vi "MD420_ACT_TargetValue-LAPTOP-A1ILEVN9.vi"(0 "MD420.lvclass":refnum<class "MD420.lvclass">, 1 "SI656 PG 2nd Min in %":dbl, 2 "SI657 PG target SP":dbl, 3 "BC56 PUMA RELEB":bool, 4 "SI101 ACT 2nd Ctrl":dbl, 5 "error in (no error)":errorcluster, 6 "SI657 PG eff SP":dbl, 7 "ACT limit Setpoint":dbl) -> (14 "MD420.lvclass out":refnum<class "MD420.lvclass">, 16 "Outputs":T1, 19 "error out":errorcluster)   [LabVIEW 2022 SP3, in "MD420.lvclass"]
uses:
  MD420.lvclass
  MD420.lvclass/MD420.ctl
panel:
  in  "H 2":dbl=22.0 format="%#_13g"
  in  "Min":dbl=26.0 format="%#_13g"
  in  "Max":dbl=26.0 format="%#_13g"
  in  "H":dbl=22.0 format="%#_13g"
  # "MD420"
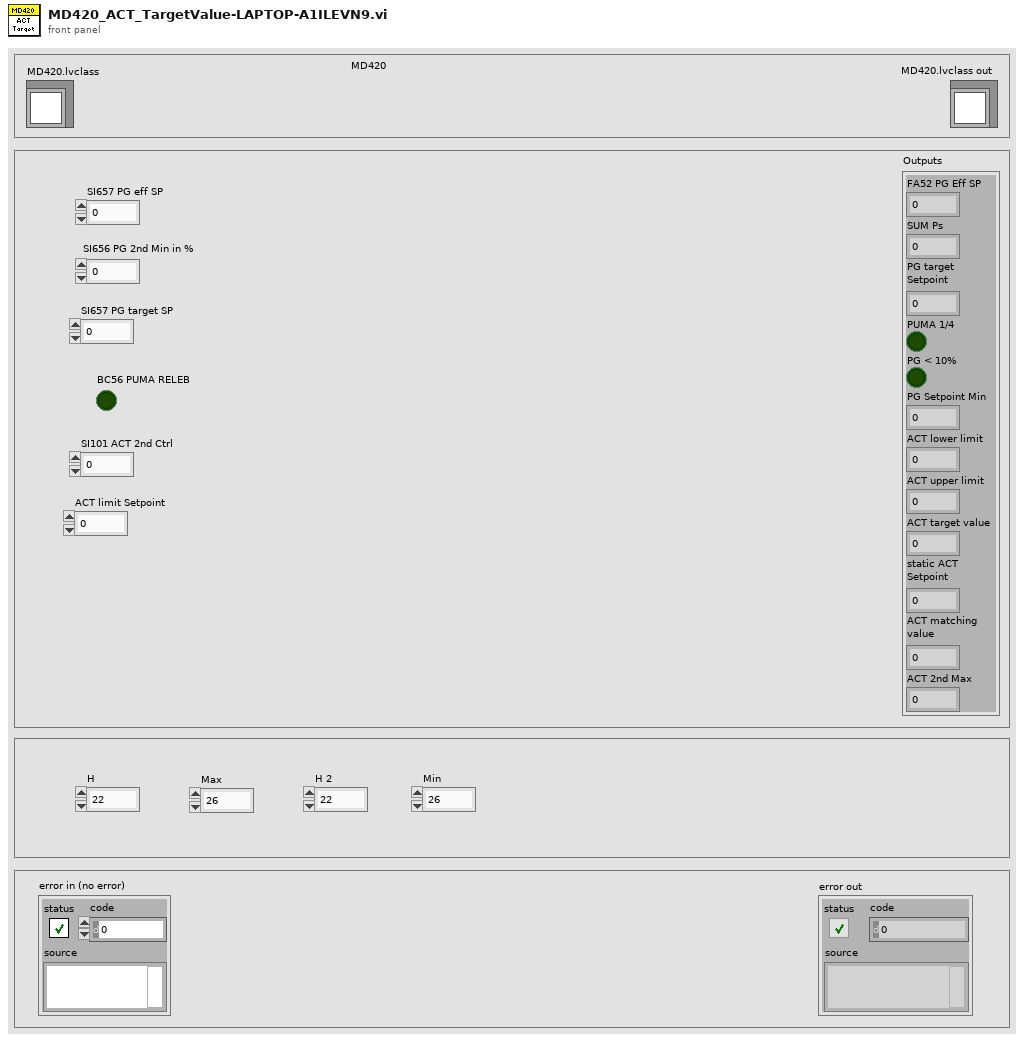
[diagram p1: front panel]
types:
  T1 = cluster{"FA52 PG Eff SP":dbl, "SUM Ps":dbl, "PG target\nSetpoint":dbl, "PUMA 1/4":bool, "PG < 10%":bool, "PG Setpoint Min":dbl, "ACT lower limit":dbl, "ACT upper limit":dbl, "ACT target value":dbl, "static ACT\nSetpoint":dbl, "ACT matching\nvalue":dbl, "ACT 2nd Max":dbl}
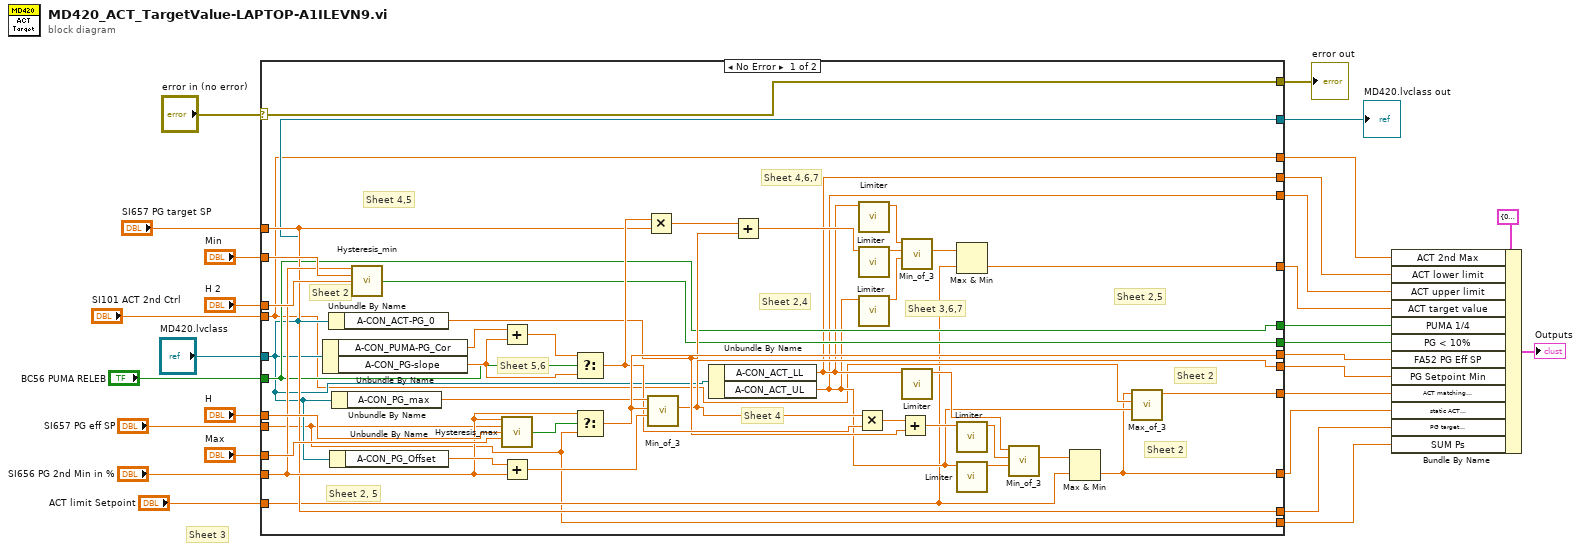
[diagram p0: block diagram]
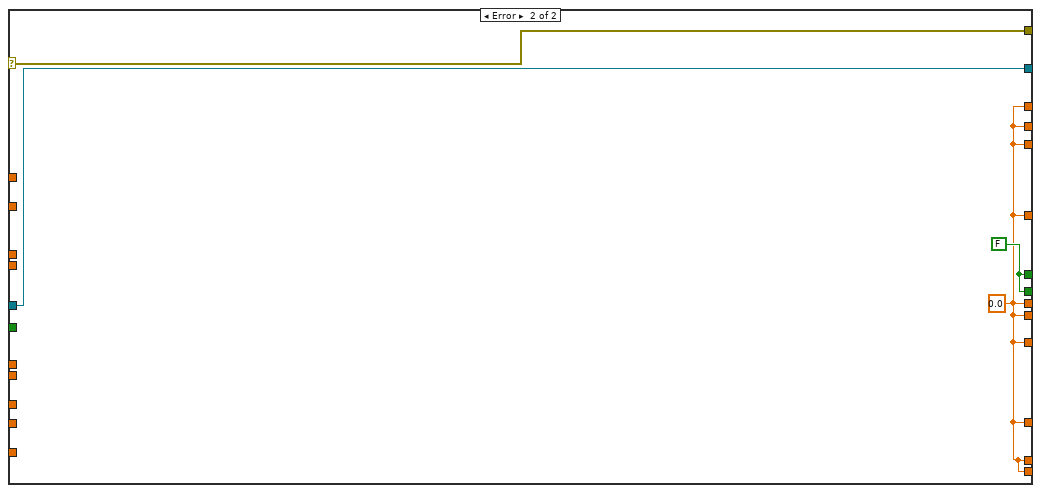
[diagram p2: hidden frame]
diagram:
  # "Sheet 3"
  n1 = case shown="No Error" "error in (no error)" {
    selector: "error in (no error)" -> [w69 w73]
    tunnel: [w69 w73] -> w27
    tunnel: "MD420.lvclass" -> [w47 w71]
    tunnel: "SI657 PG eff SP" -> [w29 _]
    tunnel: "SI656 PG 2nd Min in %" -> [w62 _]
    tunnel: "H" -> [w68 _]
    tunnel: "Max" -> [w67 _]
    tunnel: [w61 w70] -> w6
    tunnel: "Min" -> [w64 _]
    tunnel: "H 2" -> [w63 _]
    tunnel: "SI657 PG target SP" -> [w51 _]
    tunnel: "BC56 PUMA RELEB" -> [w50 _]
    tunnel: [w51 w70] -> w2
    tunnel: [w50 w72] -> w8
    tunnel: [w49 w72] -> w7
    tunnel: [w48 w70] -> w5
    tunnel: [w41 w70] -> w11
    tunnel: [w37 w70] -> w10
    tunnel: [w47 w71] -> w17
    tunnel: [w31 w70] -> w9
    tunnel: [w32 w70] -> w3
    tunnel: "SI101 ACT 2nd Ctrl" -> [w35 _]
    tunnel: [w36 w70] -> w4
    tunnel: [w35 w70] -> w12
    tunnel: "ACT limit Setpoint" -> [w30 _]
    tunnel: [w29 w70] -> w1
    frame No Error {
      # "Sheet 2"
      # "Sheet 2"
      # "Sheet 2,5"
      # "Sheet 2"
      # "Sheet 3,6,7"
      # "Sheet 4,6,7"
      # "Sheet 4"
      # "Sheet 5,6"
      # "Sheet 2,4"
      # "Sheet 4,5"
      # "Sheet 2, 5"
      n2 = Unbundle By Name(w47) -> ("A-CON_PUMA-PG_Cor"=w58:dbl, "A-CON_PG-slope"=w56:dbl)
      n3 = Unbundle By Name(w47) -> ("A-CON_ACT-PG_0"=w54:dbl)
      n4 = Unbundle By Name(w47) -> ("A-CON_PG_Offset"=w65:dbl)
      n5 = Unbundle By Name(w47) -> ("A-CON_PG_max"=w59:dbl)
      n6 = call "Hysteresis_min.vi"("input"=w62, "Min"=w64, "H"=w63) -> ("Deviation"=w49:bool)  [unwired: 11 in, 1 out]
      n7 = Add(x=w58, y=w56) -> (x+y=w57:dbl)
      n8 = call "Hysteresis_max.vi"("input(+)"=w62, "input (-)"=w29, "H"=w68, "Max"=w67) -> ("Deviation"=w66:bool)  [unwired: 10 in, 1 out]
      n9 = Add(x=w65, y=w62) -> (x+y=w60:dbl)
      n10 = Select(t=w57, s=w50, f=w56) -> (s? t:f=w55:dbl)
      n11 = Select(t=w62, s=w66, f=w29) -> (s? t:f=w61:dbl)
      n12 = Multiply(x=w55, y=w51) -> (x*y=w52:dbl)
      n13 = call "Min_of_3.vi"("input 02"=w60, "input 01"=w61, "input 03"=w59) -> ("min"=w48:dbl)  [unwired: 7 in, 1 out]
      n14 = Unbundle By Name(w47) -> ("A-CON_ACT_LL"=w41:dbl, "A-CON_ACT_UL"=w37:dbl)
      n15 = Add(x=w52, y=w54) -> (x+y=w43:dbl)
      n16 = Multiply(x=w48, y=w55) -> (x*y=w53:dbl)
      n17 = call "Limiter.vi"("input"=w41) -> ("LIMITER_PG_lift-up.UL out"=w40:dbl)  [unwired: 9 in, 1 out]
      n18 = call "Limiter.vi"("input"=w43) -> ("LIMITER_PG_lift-up.UL out"=w39:dbl)  [unwired: 9 in, 1 out]
      n19 = call "Limiter.vi"("input"=w37) -> ("LIMITER_PG_lift-up.UL out"=w38:dbl)  [unwired: 9 in, 1 out]
      n20 = Add(x=w53, y=w54) -> (x+y=w42:dbl)
      n21 = call "Min_of_3.vi"("input 02"=w38, "input 01"=w39, "input 03"=w40) -> ("min"=w33:dbl)  [unwired: 7 in, 1 out]
      n22 = call "Limiter.vi"("input"=w41) -> ("LIMITER_PG_lift-up.UL out"=w46:dbl)  [unwired: 9 in, 1 out]
      n23 = Max & Min(x=w33, y=w30) -> (min(x,y)=w31:dbl)  [unwired: 1 out]
      n24 = call "Limiter.vi"("input"=w42) -> ("LIMITER_PG_lift-up.UL out"=w45:dbl)  [unwired: 9 in, 1 out]
      n25 = call "Limiter.vi"("input"=w37) -> ("LIMITER_PG_lift-up.UL out"=w44:dbl)  [unwired: 9 in, 1 out]
      n26 = call "Min_of_3.vi"("input 02"=w44, "input 01"=w45, "input 03"=w46) -> ("min"=w34:dbl)  [unwired: 7 in, 1 out]
      n27 = Max & Min(x=w34, y=w30) -> (min(x,y)=w32:dbl)  [unwired: 1 out]
      n28 = call "Max_of_3.vi"("input 2"=w37, "input 3"=w35, "input 1"=w32) -> ("Numeric out"=w36:dbl)  [unwired: 7 in, 1 out]
    }
    frame Error {
      w70 = 0.0 ("A-CON_ACT_LL")
      w72 = FALSE ("Deviation")
    }
  }
  "error out" <- w27
  "MD420.lvclass out" <- w17
  n29 = Bundle By Name(cluster=T1 {"FA52 PG Eff SP"=0.0, "SUM Ps"=0.0, "PG target\nSetpoint"=0.0, "PUMA 1/4"=FALSE, "PG < 10%"=FALSE, "PG Setpoint Min"=0.0, "ACT lower limit"=0.0, "ACT upper limit"=0.0, "ACT target value"=0.0, "static ACT\nSetpoint"=0.0, "ACT matching\nvalue"=0.0, "ACT 2nd Max"=0.0} ("Outputs"), "ACT 2nd Max"=w12, "ACT lower limit"=w11, "ACT upper limit"=w10, "ACT target value"=w9, "PUMA 1/4"=w8, "PG < 10%"=w7, "FA52 PG Eff SP"=w6, "PG Setpoint Min"=w5, "ACT matching\nvalue"=w4, "static ACT\nSetpoint"=w3, "PG target\nSetpoint"=w2, "SUM Ps"=w1) -> (→"Outputs":T1)
